vi "CalcBGDuration.vi"(8 "Wait":i32=3 min=0 step=1, 9 "Cycle time\n(ms)":i32=3 min=0 step=1, 10 "# Frames":i32=1000 min=0 step=1, 11 "MODE":u16(ring) items=["Normal", "DIF"]) -> (3 "Duration (ms)":i32)   [LabVIEW 2018]
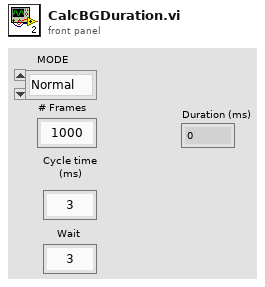
[diagram p1: front panel]
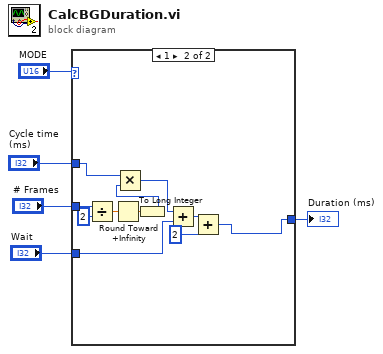
[diagram p0: block diagram]
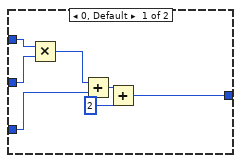
[diagram p2: hidden frame]
diagram:
  n1 = case shown="1" "MODE" {
    tunnel: "# Frames" -> [w11 w17]
    tunnel: "Cycle time\n(ms)" -> [w12 w20]
    tunnel: "Wait" -> [w10 w19]
    tunnel: [w6 w18] -> w1
    frame 0, Default {
      n2 = Multiply(x=w12, y=w11) -> (x*y=w9:i32)
      n3 = Add(x=w9, y=w10) -> (x+y=w8:i32)
      n4 = Add(x=w8, y=2) -> (x+y=w6:i32)
    }
    frame 1 {
      n5 = Divide(x=w17, y=2) -> (x/y=w15:dbl)
      n6 = Round Toward +Infinity(x=w15) -> (ceil(x): smallest int >= x=w14:dbl)
      n7 = To Long Integer(number=w14) -> (32bit integer=w13:i32)
      n8 = Multiply(x=w20, y=w13) -> (x*y=w23:i32)
      n9 = Add(x=w23, y=w19) -> (x+y=w22:i32)
      n10 = Add(x=w22, y=2) -> (x+y=w18:i32)
    }
  }
  "Duration (ms)" <- w1
